vi "getTerminalBounds.VI"(8 "Permutation":i16, 11 "Pattern":i16) -> (2 "Terminal Bounds[]":T1[](array[typedef]))   [LabVIEW 2020]
uses:
  <vilib>/Utility/miscctls.llb/LVRectTypeDef.ctl
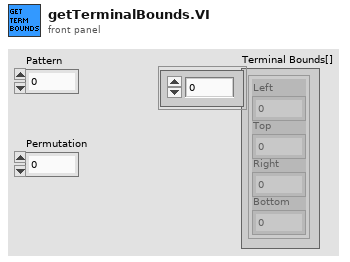
[diagram p1: front panel]
types:
  T1 = typedef "LVRectTypeDef.ctl" = cluster{"Left":i16, "Top":i16, "Right":i16, "Bottom":i16}
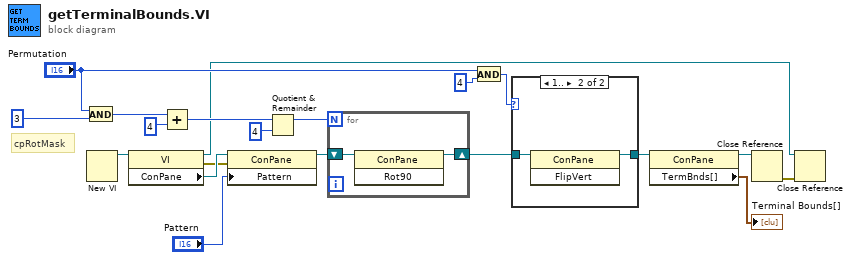
[diagram p0: block diagram]
diagram:
  # "cpRotMask"
  n1 = And(x="Permutation", y=i16 3) -> (x .and. y?=w13:i16)
  n2 = New VI() -> (3:w20:refnum<vi>)  [unwired: 7 in, 1 out]
  n3 = property class="VI"(reference=w20) -> (reference out=w1:refnum<vi>, error out=w17:errorcluster, "ConPane"=w18:refnum<vi>)  [unwired: 1 in]
  n4 = Add(x=w13, y=i16 4) -> (x+y=w11:i16)
  n5 = property class="ConPane"(reference=w18, error in=w17, "Pattern"="Pattern") -> (reference out=w8:refnum<vi>)  [unwired: 1 out]
  n6 = Quotient & Remainder(x=w11, y=i16 4) -> (x-y*floor(x/y)=w9:i16)  [unwired: 1 out]
  n7 = for {
    N: w9 -> [_]
    shift-right: [w21] -> w7
    shift-left: w8 -> [w22]
    n8 = invoke class="ConPane" method="Rot90"(reference=w22) -> (reference out=w21:refnum<vi>)  [unwired: 2 in, 2 out]
  }
  n9 = And(x="Permutation", y=i16 4) -> (x .and. y?=w6:i16)
  n10 = case shown="1.." w6 {
    tunnel: w7 -> [w23 w25]
    tunnel: [w23 w24] -> w5
    frame 0, Default {
    }
    frame 1.. {
      n11 = invoke class="ConPane" method="FlipVert"(reference=w25) -> (reference out=w24:refnum<vi>)  [unwired: 2 in, 2 out]
    }
  }
  n12 = property class="ConPane"(reference=w5) -> (reference out=w3:refnum<vi>, "TermBnds[]"=→"Terminal Bounds[]":T1[])  [unwired: 1 in, 1 out]
  n13 = Close Reference(reference=w3) -> (error out=w2:errorcluster)  [unwired: 1 in]
  n14 = Close Reference(reference=w1, error in (no error)=w2) -> ()  [unwired: 1 out]
